vi "Served_Global.vi"(0 "Mode":T1) -> (1 "Served VI Name":string[](array[string]), 2 "Served VI Path":path[](array[path]), 3 "Served IP Number & Port No":string[](array[string]))   [LabVIEW 2020]
uses:
  Controls/Serveds.ctl
  File/Setup_Filetype.ctl
  Preference_global.vi
  Constants_global.vi
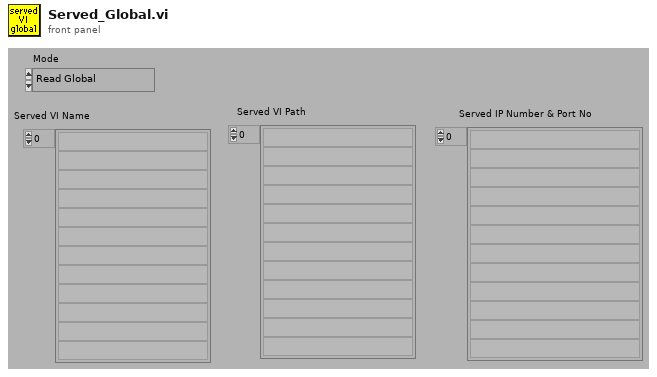
[diagram p1: front panel]
types:
  T1 = typedef "Serveds.ctl" = enum16{"Read Global", "Load Global From File"}
  T2 = typedef "Setup_Filetype.ctl" = enum16{"Measurement Setups", "Calibration Setups", "General", "Results File Plotter Setups", "Speed Calib Tweaks"}
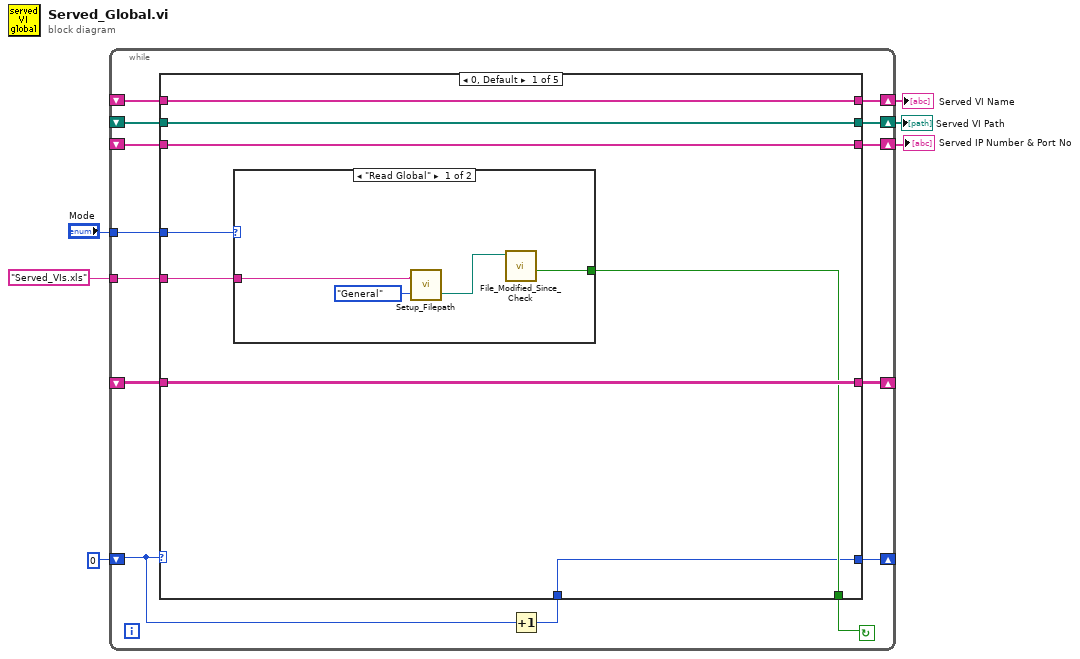
[diagram p0: block diagram]
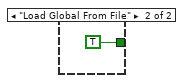
[diagram p2: hidden frame]
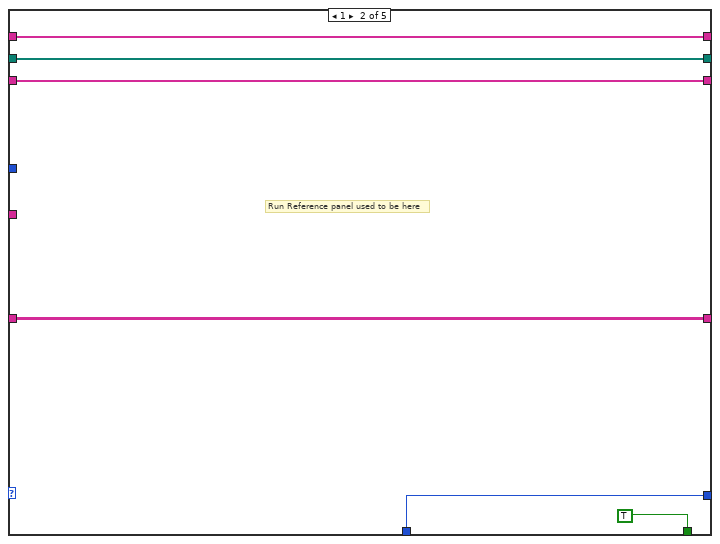
[diagram p3: hidden frame]
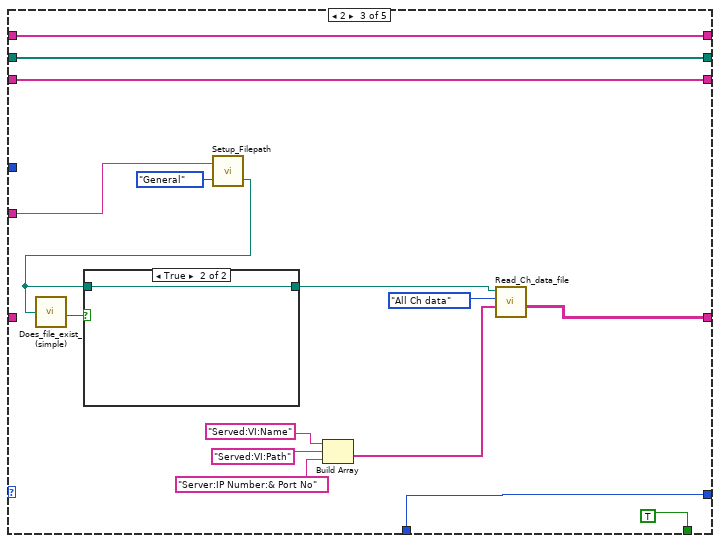
[diagram p4: hidden frame]
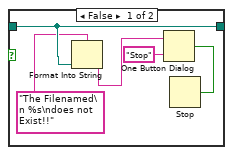
[diagram p5: hidden frame]
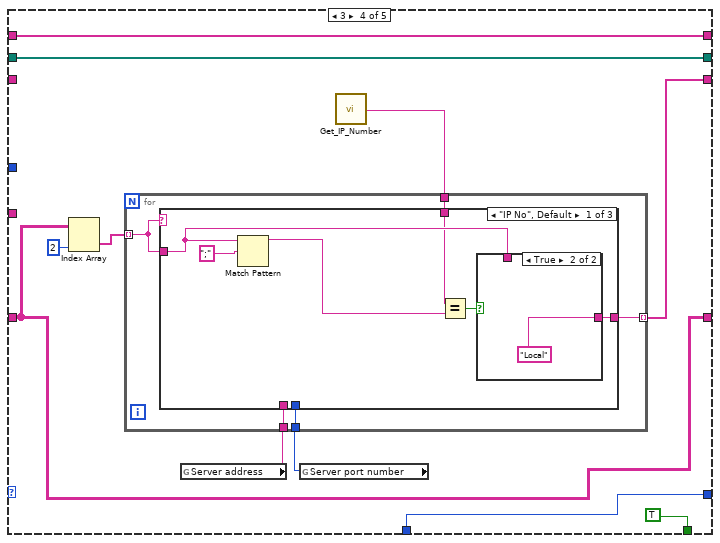
[diagram p6: hidden frame]
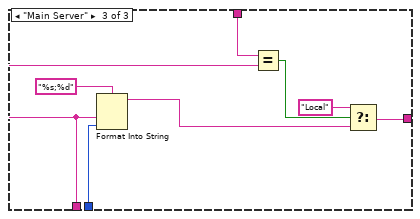
[diagram p9: hidden frame]
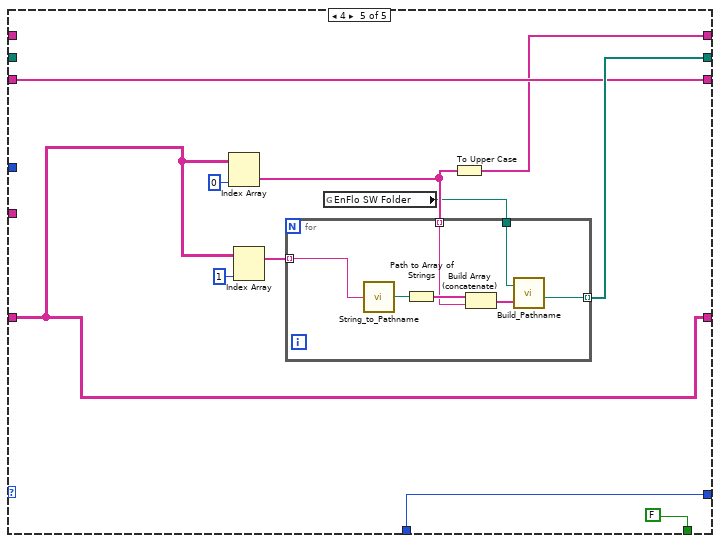
[diagram p10: hidden frame]
diagram:
  n1 = while {
    shift-left: _ -> [w8]
    shift-right: [w13] -> w4
    shift-left: _ -> [w12]
    shift-right: [w11] -> w3
    shift-left: _ -> [w10]
    shift-right: [w9] -> w2
    shift-left: _ -> [w16]
    shift-right: [w17] -> _
    tunnel: "Mode" -> [w18]
    shift-left: 0 -> [w15]
    shift-right: [w19] -> _
    tunnel: "Served_VIs.xls" ("Substring") -> [w7]
    stop <- w20 continue-if-true
    n2 = Increment(x=w15) -> (x+1=w14:i32)
    n3 = case shown="0, Default" w15 {
      tunnel: [w26 TRUE TRUE TRUE FALSE] -> w20
      tunnel: [w25 w37 w50 w69 w104] -> w19
      tunnel: w18 -> [w27 _ _ _ _]
      tunnel: [w28 w39 w53 w66 w98] -> w17
      tunnel: w16 -> [w28 w39 _ w66 w98]
      tunnel: w14 -> [w25 w37 w50 w69 w104]
      tunnel: [w22 w34 w43 w67 w100] -> w13
      tunnel: w12 -> [w23 w35 w44 w64 _]
      tunnel: [w23 w35 w44 w64 w101] -> w11
      tunnel: w10 -> [w24 w36 w45 w63 _]
      tunnel: [w24 w36 w45 w63 w95] -> w9
      tunnel: w8 -> [w22 w34 w43 _ w100]
      tunnel: w7 -> [w21 _ w41 _ _]
      frame 0, Default {
        n4 = case shown="\"Read Global\"" w27 {
          tunnel: [w29 TRUE ("Modified?")] -> w26
          tunnel: w21 -> [w31 _]
          frame "Read Global" {
            n5 = call "Setup_Filepath.vi"("Setup File Type"=Setup_Filetype."General", "Filename in"=w31) -> ("Filename Out"=w30:path)  [unwired: 1 out]
            n6 = call "File_Modified_Since_Check.vi"("File Path"=w30) -> ("modifiedSinceRead"=w29:bool)  [unwired: 7 in, 1 out]
          }
          frame "Load Global From File" {
          }
        }
      }
      frame 1 {
        # "Run Reference panel used to be here"
      }
      frame 2 {
        n7 = call "Setup_Filepath.vi"("Setup File Type"=Setup_Filetype."General", "Filename in"=w41) -> ("Filename Out"=w40:path)  [unwired: 1 out]
        n8 = call "Does_file_exist_(simple).vi"("Pathname"=w40) -> ("exists?"=w52:bool)
        n9 = case shown="True" w52 {
          tunnel: w40 -> [w57 w61]
          tunnel: [w57 w61] -> w51
          frame False {
            n10 = Format Into String(format string="The Filenamed\n %s\ndoes not Exist!!" ("Format String"), w57) -> (resulting string=w59:string)  [unwired: 2 in, 1 out]
            n11 = One Button Dialog(message=w59, button name ("OK")="Stop") -> (true=w58:bool)
            n12 = Stop(stop? (T)=w58) -> ()
          }
          frame True {
          }
        }
        n13 = Build Array("Served:VI:Name", "Served:VI:Path", "Server:IP Number:& Port No") -> (w46:string[])
        n14 = call "Read_Ch_data_file.vi"("Present Channels"=w46, "Output"=enum16{"All Ch data", "The last few rows"}."All Ch data", "Filename"=w51) -> ("Channel Values"=w53:string[][])  [unwired: 2 in, 4 out]
      }
      frame 3 {
        n15 = Index Array(array=w66, index (col)=2) -> (element=w65:string[])  [unwired: 1 in]
        n16 = global read "Preference_global.vi" "Server address"() -> (w71:string)
        n17 = global read "Preference_global.vi" "Server port number"() -> (w70:u32)
        n18 = call "Get_IP_Number.vi"() -> ("IP Number"=w62:string)  [unwired: 1 out]
        n19 = for {
          tunnel: [w77] -> w67 mode=indexing
          tunnel: w71 -> [w76]
          tunnel: w70 -> [w75]
          tunnel: w62 -> [w74]
          tunnel: w65 -> [w73] mode=indexing
          n20 = case shown="\"IP No\", Default" w73 {
            tunnel: [w82 w86 w87] -> w77
            tunnel: w76 -> [_ _ w91]
            tunnel: w75 -> [_ _ w94]
            tunnel: w73 -> [w80 w86 _]
            tunnel: w74 -> [w78 _ w92]
            frame "IP No", Default {
              n21 = Match Pattern(string=w80, regular expression=";") -> (before substring=w79:string)  [unwired: 4 out]
              n22 = Equal?(x=w78, y=w79) -> (x = y?=w81:bool)
              n23 = case shown="True" w81 {
                tunnel: [w84 "Local" ("t")] -> w82
                tunnel: w80 -> [w84 _]
                frame False {
                }
                frame True {
                }
              }
            }
            frame "Local" {
            }
            frame "Main Server" {
              n24 = Format Into String(format string="%s;%d" ("Format String"), w91, w94) -> (resulting string=w89:string)  [unwired: 2 in, 1 out]
              n25 = Equal?(x=w92, y=w91) -> (x = y?=w90:bool)
              n26 = Select(t="Local", s=w90, f=w89) -> (s? t:f=w87:string)
            }
          }
        }
      }
      frame 4 {
        n27 = Index Array(array=w98, index (col)=0 ("Index")) -> (element=w97:string[])  [unwired: 1 in]
        n28 = Index Array(array=w98, index (col)=1 ("Index")) -> (element=w102:string[])  [unwired: 1 in]
        n29 = global read "Constants_global.vi" "EnFlo SW Folder"() -> (w96:path)
        n30 = for {
          tunnel: w102 -> [w112] mode=indexing
          tunnel: [w106] -> w101 mode=indexing
          tunnel: w97 -> [w109] mode=indexing
          tunnel: w96 -> [w108]
          n31 = call "String_to_Pathname.vi"("Input String"=w112) -> ("path"=w111:path)
          n32 = Path to Array of Strings(0:w111) -> (2:w110:string[])  [unwired: 1 out]
          n33 = Build Array (concatenate)(w110, w109) -> (w107:string[])
          n34 = call "Build_Pathname.vi"("PathElements"=w107, "PathnameIn"=w108) -> ("AppendedPath"=w106:path)
        }
        n35 = To Upper Case(1:w97) -> (0:w95:string[])
      }
    }
  }
  "Served IP Number & Port No" <- w4
  "Served VI Name" <- w2
  "Served VI Path" <- w3
